vi "get_id_string.vi"(8 "error in (no error)":errorcluster, 11 "Modbus Master in":refnum<class "Modbus Master.lvclass">) -> (0 "error out":errorcluster, 2 "ID String":string, 3 "Modbus Master out":refnum<class "Modbus Master.lvclass">)   [LabVIEW 2018]
uses:
  <vilib>/NI/Modbus Library/API/Master/Modbus Master.lvclass
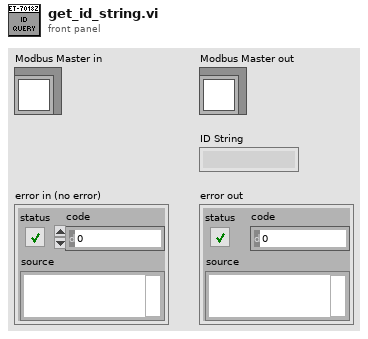
[diagram p1: front panel]
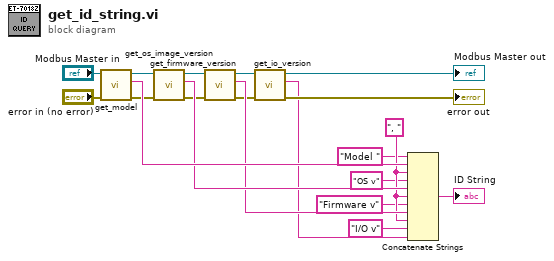
[diagram p0: block diagram]
diagram:
  w9 = ", " ("string")
  n1 = call "get_model.vi"("error in (no error)"="error in (no error)", "Modbus Master in"="Modbus Master in") -> ("error out"=w18:errorcluster, "Model"=w20:string, "Modbus Master out"=w19:refnum<class "Modbus Master.lvclass">)  [unwired: 7 in]
  n2 = call "get_os_image_version.vi"("error in (no error)"=w18, "Modbus Master in"=w19) -> ("error out"=w2:errorcluster, "OS image version"=w12:string, "Modbus Master out"=w1:refnum<class "Modbus Master.lvclass">)  [unwired: 7 in]
  n3 = call "get_firmware_version.vi"("error in (no error)"=w2, "Modbus Master in"=w1) -> ("error out"=w4:errorcluster, "Firmware version"=w11:string, "Modbus Master out"=w3:refnum<class "Modbus Master.lvclass">)  [unwired: 7 in]
  n4 = call "get_io_version.vi"("error in (no error)"=w4, "Modbus Master in"=w3) -> ("error out"=→"error out":errorcluster, "I/O version"=w10:string, "Modbus Master out"=→"Modbus Master out":refnum<class "Modbus Master.lvclass">)  [unwired: 7 in]
  n5 = Concatenate Strings("Model " ("string"), w20, w9, "OS v" ("string"), w12, w9, "Firmware v" ("string"), w11, w9, "I/O v" ("string"), w10) -> (→"ID String":string)
